vi "amy_test.vi"() -> ()   [LabVIEW 2017]
panel:
  in  "Filename":path=path "amy_test.xlsx"
  out "Waveform Graph":dynamicdata(graph)
  in  "stop 2":bool
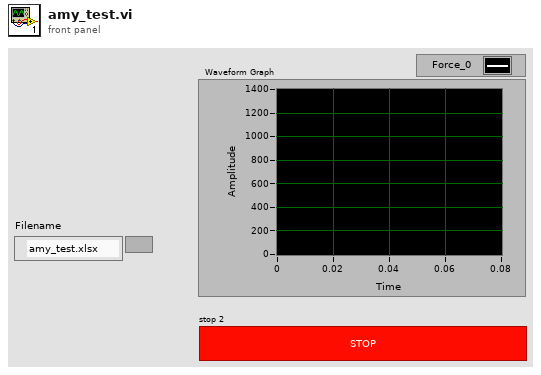
[diagram p1: front panel]
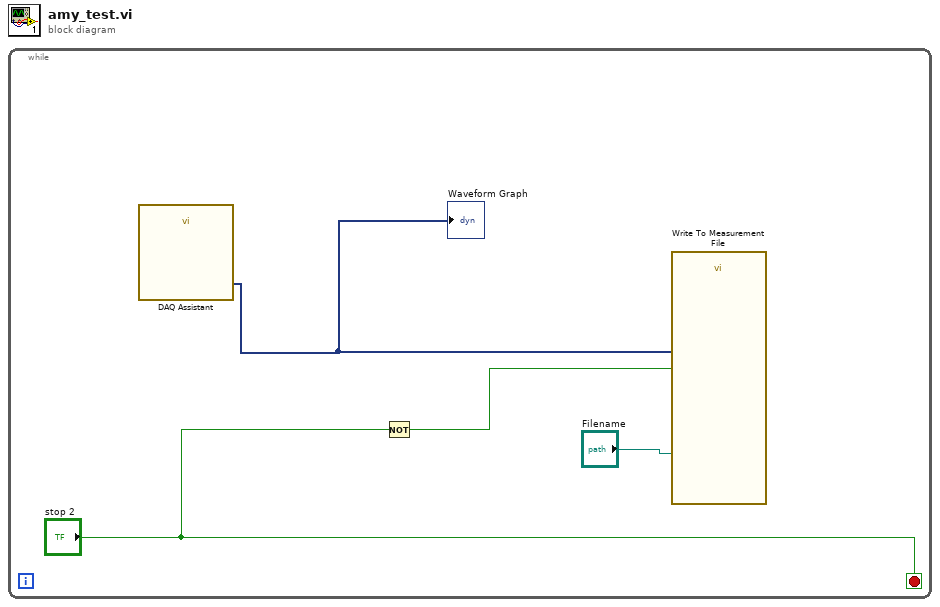
[diagram p0: block diagram]
diagram:
  n1 = while {
    stop <- "stop 2" stop-if-true
    n2 = call "DAQ Assistant"() -> ("data"=w2:dynamicdata)  [unwired: 17 in, 2 out]
    "Waveform Graph" <- w2
    n3 = Not(x="stop 2") -> (.not. x?=w4:bool)
    n4 = call "Write To Measurement File"("Signals"=w2, "Flush? (T)"=w4, "Filename"="Filename") -> ()  [unwired: 14 in, 3 out]
  }
